vi "Encoders Read.vi"(6 "Motors Renum":cluster{"Num":i32, "Directly":bool, "KM":dbl}[](array[cluster]), 8 "error in (no error)":errorcluster, 9 "Start":bool, 11 "TitanENC in":T4) -> (0 "error out":errorcluster, 1 "ENC True":T2, 2 "ENC":T2, 3 "TitanENC out":T5, 4 "RPM":T1, 5 "ENC/dt":T3)   [LabVIEW 2020]
uses:
  <vilib>/High Genius/HG_WSI_Tookit/Dependencies/Library/TitanENC/TitanENC.lvclass
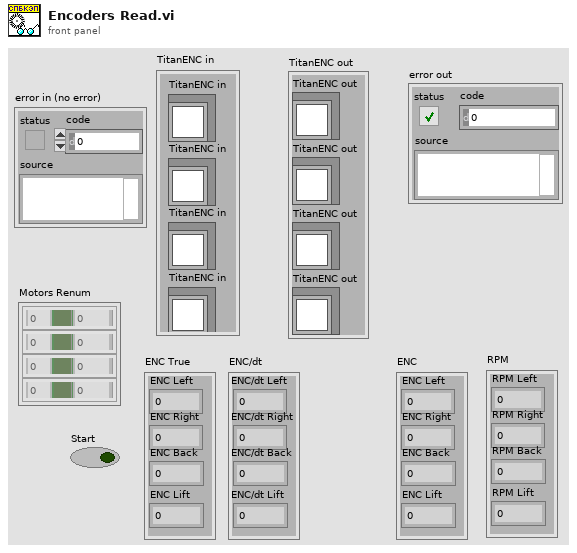
[diagram p1: front panel]
types:
  T1 = cluster{"RPM Left":i32, "RPM Right":i32, "RPM Back":i32, "RPM Lift":i32}
  T2 = cluster{"ENC Left":i32, "ENC Right":i32, "ENC Back":i32, "ENC Lift":i32}
  T3 = cluster{"ENC/dt Left":i32, "ENC/dt Right":i32, "ENC/dt Back":i32, "ENC/dt Lift":i32}
  T4 = cluster{"TitanENC in":refnum<class "TitanENC.lvclass">, "TitanENC in":refnum<class "TitanENC.lvclass">, "TitanENC in":refnum<class "TitanENC.lvclass">, "TitanENC in":refnum<class "TitanENC.lvclass">}
  T5 = cluster{"TitanENC out":refnum<class "TitanENC.lvclass">, "TitanENC out":refnum<class "TitanENC.lvclass">, "TitanENC out":refnum<class "TitanENC.lvclass">, "TitanENC out":refnum<class "TitanENC.lvclass">}
  T6 = cluster{"titanenc0":i32, "titanenc1":i32, "titanenc2":i32, "titanenc3":i32, "rpm0":i16, "rpm1":i16, "rpm2":i16, "rpm3":i16, "resetenc0":bool, "resetenc1":bool, "resetenc2":bool, "resetenc3":bool}
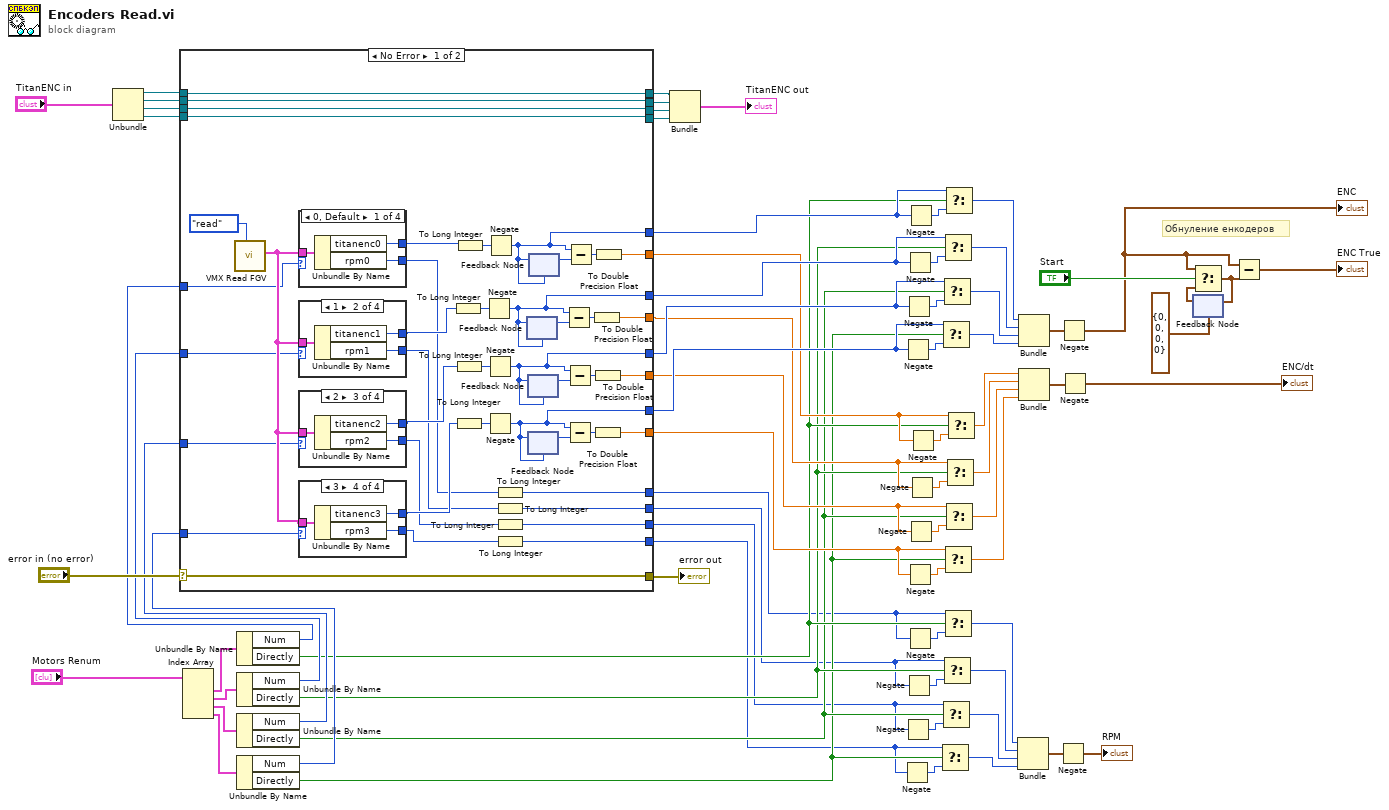
[diagram p0: block diagram]
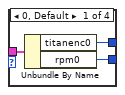
[diagram p2: hidden frame]
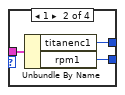
[diagram p3: hidden frame]
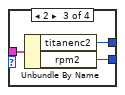
[diagram p4: hidden frame]
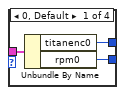
[diagram p5: hidden frame]
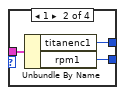
[diagram p6: hidden frame]
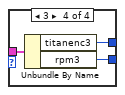
[diagram p7: hidden frame]
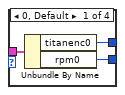
[diagram p8: hidden frame]
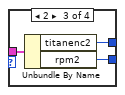
[diagram p9: hidden frame]
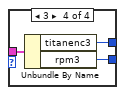
[diagram p10: hidden frame]
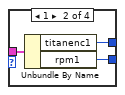
[diagram p11: hidden frame]
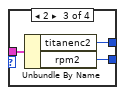
[diagram p12: hidden frame]
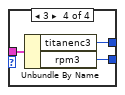
[diagram p13: hidden frame]
diagram:
  # "Обнуление енкодеров"
  n1 = Unbundle("TitanENC in") -> ("TitanENC in"=w72:refnum<class "TitanENC.lvclass">, "TitanENC in"=w71:refnum<class "TitanENC.lvclass">, "TitanENC in"=w70:refnum<class "TitanENC.lvclass">, "TitanENC in"=w69:refnum<class "TitanENC.lvclass">)
  n2 = Index Array(array="Motors Renum") -> (element #1=w51:cluster{"Num":i32, "Directly":bool, "KM":dbl}, element #2=w50:cluster{"Num":i32, "Directly":bool, "KM":dbl}, element #3=w49:cluster{"Num":i32, "Directly":bool, "KM":dbl}, element #4=w48:cluster{"Num":i32, "Directly":bool, "KM":dbl})  [unwired: 4 in]
  n3 = Unbundle By Name(w51) -> ("Num"=w22:i32, "Directly"=w8:bool)
  n4 = Unbundle By Name(w50) -> ("Num"=w21:i32, "Directly"=w7:bool)
  n5 = Unbundle By Name(w49) -> ("Num"=w20:i32, "Directly"=w6:bool)
  n6 = Unbundle By Name(w48) -> ("Num"=w19:i32, "Directly"=w5:bool)
  n7 = case shown="No Error" "error in (no error)" {
    selector: "error in (no error)" -> [w115 w168]
    tunnel: [w115 w168] -> w62
    tunnel: [w114 w167] -> w67
    tunnel: w72 -> [w114 w167]
    tunnel: [w113 w166] -> w66
    tunnel: [w112 w165] -> w65
    tunnel: [w111 w164] -> w64
    tunnel: w71 -> [w113 w166]
    tunnel: w70 -> [w112 w165]
    tunnel: w69 -> [w111 w164]
    tunnel: [w97 _] -> w43
    tunnel: [w93 _] -> w42
    tunnel: [w92 _] -> w41
    tunnel: [w91 _] -> w40
    tunnel: [w98 _] -> w31
    tunnel: [w96 _] -> w30
    tunnel: [w95 _] -> w29
    tunnel: [w94 _] -> w28
    tunnel: w22 -> [w84 _]
    tunnel: w21 -> [w83 _]
    tunnel: w20 -> [w82 _]
    tunnel: w19 -> [w81 _]
    tunnel: [w76 _] -> w4
    tunnel: [w75 _] -> w3
    tunnel: [w74 _] -> w2
    tunnel: [w73 _] -> w1
    frame No Error {
      n8 = call <vilib>:"VMX Read FGV.vi"("Enum"=enum16{"read", "write"}."read") -> ("Read Data2"=w87:T6)  [unwired: 9 in, 1 out]
      n9 = case shown="0, Default" w84 {
        tunnel: w87 -> [w154 w157 w160 w163]
        tunnel: [w153 w156 w159 w162] -> w89
        tunnel: [w152 w155 w158 w161] -> w77
        frame 0, Default {
          n10 = Unbundle By Name(w154) -> ("titanenc0"=w153:i32, "rpm0"=w152:i16)
        }
        frame 1 {
          n11 = Unbundle By Name(w157) -> ("titanenc1"=w156:i32, "rpm1"=w155:i16)
        }
        frame 2 {
          n12 = Unbundle By Name(w160) -> ("titanenc2"=w159:i32, "rpm2"=w158:i16)
        }
        frame 3 {
          n13 = Unbundle By Name(w163) -> ("titanenc3"=w162:i32, "rpm3"=w161:i16)
        }
      }
      n14 = case shown="1" w83 {
        tunnel: w87 -> [w142 w145 w148 w151]
        tunnel: [w141 w144 w147 w150] -> w88
        tunnel: [w140 w143 w146 w149] -> w78
        frame 0, Default {
          n15 = Unbundle By Name(w142) -> ("titanenc0"=w141:i32, "rpm0"=w140:i16)
        }
        frame 1 {
          n16 = Unbundle By Name(w145) -> ("titanenc1"=w144:i32, "rpm1"=w143:i16)
        }
        frame 2 {
          n17 = Unbundle By Name(w148) -> ("titanenc2"=w147:i32, "rpm2"=w146:i16)
        }
        frame 3 {
          n18 = Unbundle By Name(w151) -> ("titanenc3"=w150:i32, "rpm3"=w149:i16)
        }
      }
      n19 = case shown="2" w82 {
        tunnel: w87 -> [w130 w133 w136 w139]
        tunnel: [w129 w132 w135 w138] -> w86
        tunnel: [w128 w131 w134 w137] -> w79
        frame 0, Default {
          n20 = Unbundle By Name(w130) -> ("titanenc0"=w129:i32, "rpm0"=w128:i16)
        }
        frame 1 {
          n21 = Unbundle By Name(w133) -> ("titanenc1"=w132:i32, "rpm1"=w131:i16)
        }
        frame 2 {
          n22 = Unbundle By Name(w136) -> ("titanenc2"=w135:i32, "rpm2"=w134:i16)
        }
        frame 3 {
          n23 = Unbundle By Name(w139) -> ("titanenc3"=w138:i32, "rpm3"=w137:i16)
        }
      }
      n24 = case shown="3" w81 {
        tunnel: w87 -> [w118 w121 w124 w127]
        tunnel: [w117 w120 w123 w126] -> w85
        tunnel: [w116 w119 w122 w125] -> w80
        frame 0, Default {
          n25 = Unbundle By Name(w118) -> ("titanenc0"=w117:i32, "rpm0"=w116:i16)
        }
        frame 1 {
          n26 = Unbundle By Name(w121) -> ("titanenc1"=w120:i32, "rpm1"=w119:i16)
        }
        frame 2 {
          n27 = Unbundle By Name(w124) -> ("titanenc2"=w123:i32, "rpm2"=w122:i16)
        }
        frame 3 {
          n28 = Unbundle By Name(w127) -> ("titanenc3"=w126:i32, "rpm3"=w125:i16)
        }
      }
      n29 = To Long Integer(number=w88) -> (32bit integer=w108:i32)
      n30 = To Long Integer(number=w86) -> (32bit integer=w107:i32)
      n31 = To Long Integer(number=w85) -> (32bit integer=w102:i32)
      n32 = To Long Integer(number=w89) -> (32bit integer=w99:i32)
      n33 = Negate(x=w108) -> (-x=w93:i32)
      n34 = Negate(x=w107) -> (-x=w92:i32)
      n35 = Negate(x=w102) -> (-x=w91:i32)
      n36 = Negate(x=w99) -> (-x=w97:i32)
      n37 = To Long Integer(number=w77) -> (32bit integer=w76:i32)
      n38 = To Long Integer(number=w78) -> (32bit integer=w75:i32)
      n39 = To Long Integer(number=w79) -> (32bit integer=w74:i32)
      n40 = To Long Integer(number=w80) -> (32bit integer=w73:i32)
      n41 = feedback #1(w93) -> (w110:i32)
      n42 = feedback-in #1(w93) -> ()
      n43 = feedback #2(w92) -> (w105:i32)
      n44 = feedback-in #2(w92) -> ()
      n45 = feedback #3(w91) -> (w104:i32)
      n46 = feedback-in #3(w91) -> ()
      n47 = feedback #4(w97) -> (w101:i32)
      n48 = feedback-in #4(w97) -> ()
      n49 = Subtract(x=w93, y=w110) -> (x-y=w109:i32)
      n50 = Subtract(x=w92, y=w105) -> (x-y=w106:i32)
      n51 = Subtract(x=w91, y=w104) -> (x-y=w103:i32)
      n52 = Subtract(x=w97, y=w101) -> (x-y=w100:i32)
      n53 = To Double Precision Float(number=w109) -> (double precision float=w96:dbl)
      n54 = To Double Precision Float(number=w106) -> (double precision float=w95:dbl)
      n55 = To Double Precision Float(number=w103) -> (double precision float=w94:dbl)
      n56 = To Double Precision Float(number=w100) -> (double precision float=w98:dbl)
    }
    frame Error {
    }
  }
  "error out" <- w62
  n57 = Bundle("TitanENC in"=w67, "TitanENC in"=w66, "TitanENC in"=w65, "TitanENC in"=w64) -> (→"TitanENC out":T4)  [unwired: 1 in]
  n58 = Negate(x=w1) -> (-x=w15:i32)
  n59 = Negate(x=w40) -> (-x=w45:i32)
  n60 = Negate(x=w2) -> (-x=w14:i32)
  n61 = Negate(x=w41) -> (-x=w44:i32)
  n62 = Negate(x=w3) -> (-x=w16:i32)
  n63 = Negate(x=w42) -> (-x=w46:i32)
  n64 = Negate(x=w28) -> (-x=w34:dbl)
  n65 = Negate(x=w4) -> (-x=w17:i32)
  n66 = Negate(x=w43) -> (-x=w47:i32)
  n67 = Negate(x=w29) -> (-x=w35:dbl)
  n68 = Negate(x=w30) -> (-x=w33:dbl)
  n69 = Negate(x=w31) -> (-x=w32:dbl)
  n70 = Select(t=w1, s=w5, f=w15) -> (s? t:f=w10:i32)
  n71 = Select(t=w40, s=w5, f=w45) -> (s? t:f=w36:i32)
  n72 = Select(t=w2, s=w6, f=w14) -> (s? t:f=w11:i32)
  n73 = Select(t=w41, s=w6, f=w44) -> (s? t:f=w37:i32)
  n74 = Select(t=w3, s=w7, f=w16) -> (s? t:f=w12:i32)
  n75 = Select(t=w42, s=w7, f=w46) -> (s? t:f=w38:i32)
  n76 = Select(t=w28, s=w5, f=w34) -> (s? t:f=w24:dbl)
  n77 = Select(t=w4, s=w8, f=w17) -> (s? t:f=w13:i32)
  n78 = Select(t=w43, s=w8, f=w47) -> (s? t:f=w39:i32)
  n79 = Select(t=w29, s=w6, f=w35) -> (s? t:f=w25:dbl)
  n80 = Select(t=w30, s=w7, f=w33) -> (s? t:f=w26:dbl)
  n81 = Select(t=w31, s=w8, f=w32) -> (s? t:f=w27:dbl)
  n82 = Bundle(w13, w12, w11, w10) -> (w18:cluster{i32, i32, i32, i32})  [unwired: 1 in]
  n83 = Bundle(w39, w38, w37, w36) -> (w60:cluster{i32, i32, i32, i32})  [unwired: 1 in]
  n84 = Bundle(w27, w26, w25, w24) -> (w53:cluster{dbl, dbl, dbl, dbl})  [unwired: 1 in]
  n85 = Negate(x=w18) -> (-x=→"RPM":cluster{i32, i32, i32, i32})
  n86 = Negate(x=w60) -> (-x=w55:cluster{i32, i32, i32, i32})
  "ENC" <- w55
  n87 = Negate(x=w53) -> (-x=→"ENC/dt":cluster{dbl, dbl, dbl, dbl})
  n88 = feedback #5(cluster{i32, i32, i32, i32} {0, 0, 0, 0}) -> (w58:cluster{i32, i32, i32, i32})
  n89 = Select(t=w55, s="Start", f=w58) -> (s? t:f=w59:cluster{i32, i32, i32, i32})
  n90 = feedback-in #5(w59) -> ()
  n91 = Subtract(x=w55, y=w59) -> (x-y=→"ENC True":cluster{i32, i32, i32, i32})
